vi "ManageInterfaces.vi"(0 "ClassWriterNative.lvclass":refnum<class "ClassWriterNative.lvclass">, 1 "ClassRef":refnum<vi>, 2 "HandleInterfacesData":T1, 5 "error in (no error)":errorcluster) -> (14 "ClassWriterNative.lvclass":refnum<class "ClassWriterNative.lvclass">, 19 "error out":errorcluster)   [LabVIEW 2020, in "ClassWriterNative.lvclass"]
uses:
  ClassWriterNative.lvclass
  C:/Program Files (x86)/National Instruments/LabVIEW 2020/resource/Framework/Providers/Open_GDS/ClassProviders/Provider_BaseClassInterface/ClassWriter_class/ClassWriter.lvclass
  Provider_BaseClassInterface/ClassWriter_class/HandleInterfacesData.ctl
  662f421e-4c37-4cdf-a30f-b2e85ba611a1.vi
  Common/InterfaceLibrary/InterfaceLibrary.lvlib
  Provider_BaseClassInterface/ClassWriter_class/ClassWriter.lvclass
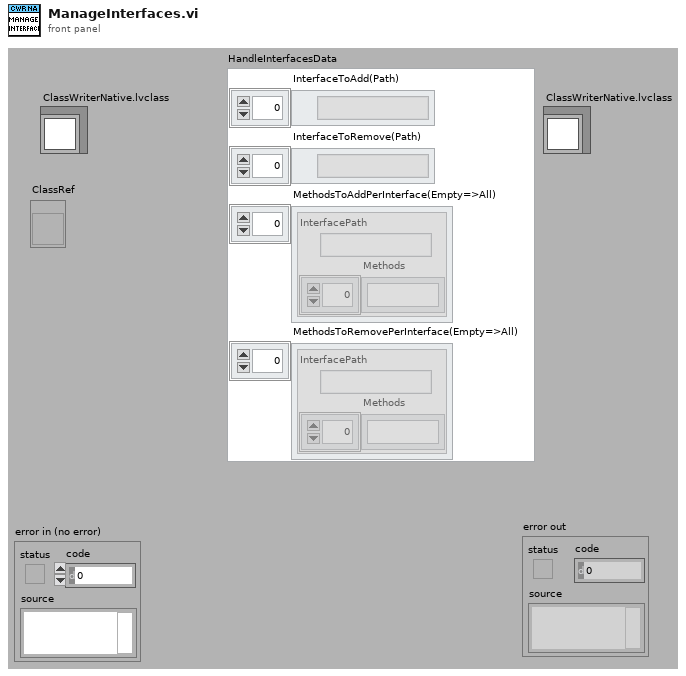
[diagram p1: front panel]
types:
  T1 = typedef "ClassWriter.lvclass/HandleInterfacesData.ctl" = cluster{"InterfaceToAdd(Path)":path[], "InterfaceToRemove(Path)":path[], "MethodsToAddPerInterface(Empty=>All)":cluster{"InterfacePath":path, "Methods":string[]}[], "MethodsToRemovePerInterface(Empty=>All)":cluster{"InterfacePath":path, "Methods":string[]}[]}
  T2 = cluster{"InterfacePath":path, "Methods":string[]}[]
  T3 = cluster{"InterfacePath":path, "Methods":string[]}
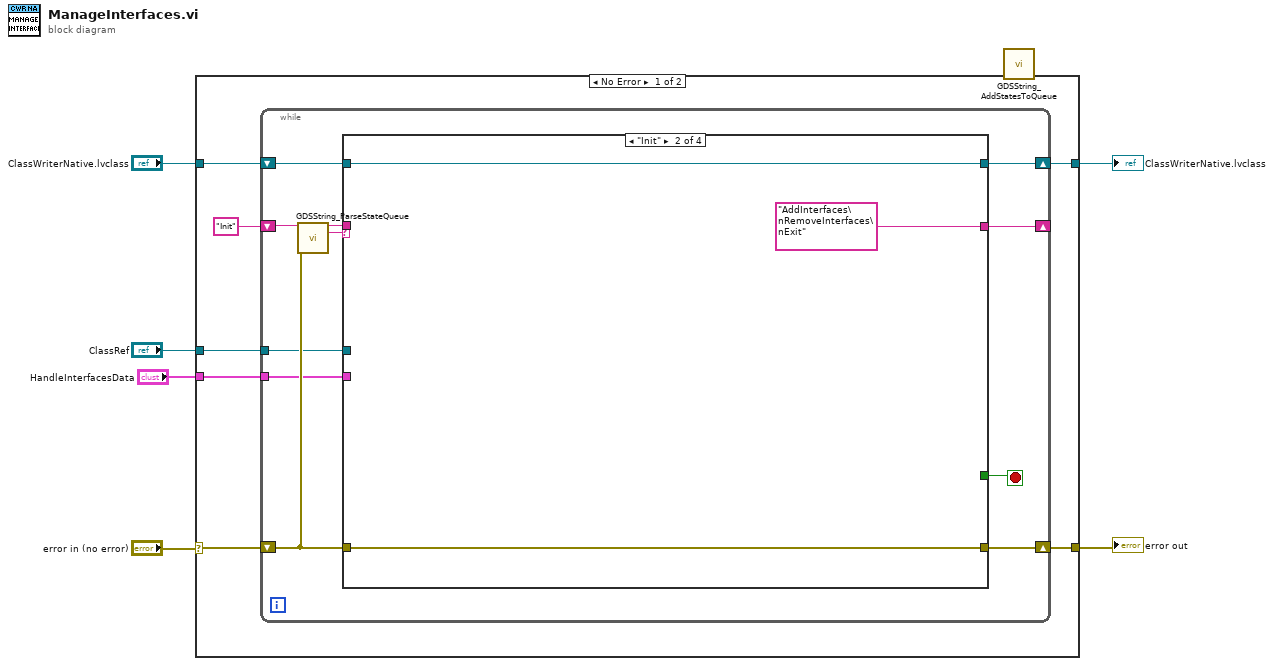
[diagram p0: block diagram]
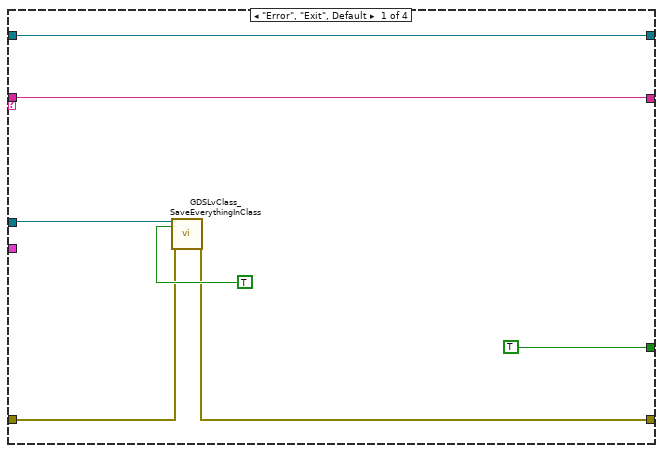
[diagram p2: hidden frame]
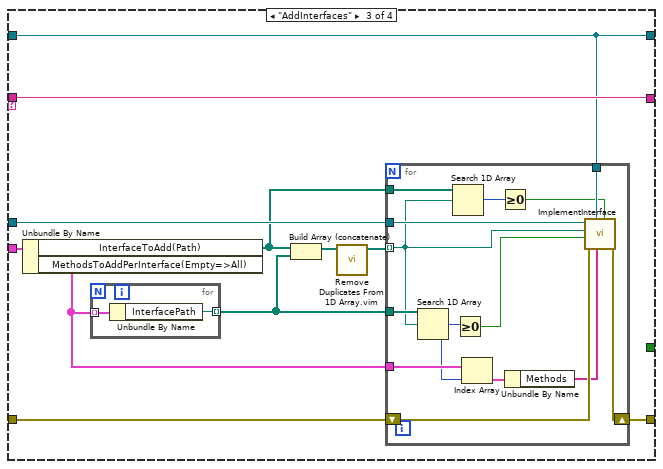
[diagram p3: hidden frame]
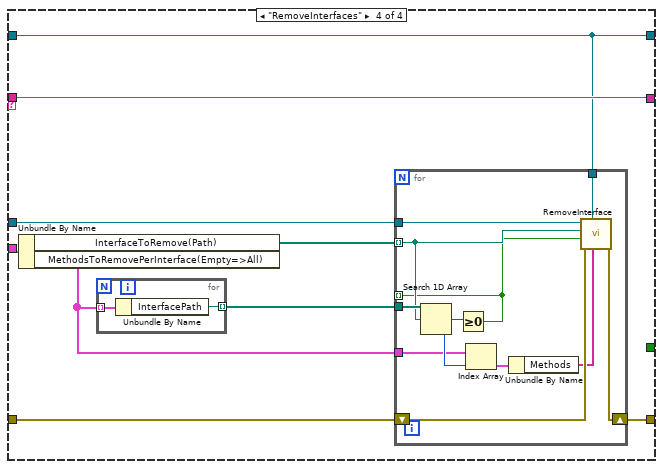
[diagram p4: hidden frame]
diagram:
  n1 = case shown="No Error" "error in (no error)" {
    selector: "error in (no error)" -> [w13 w84]
    tunnel: "ClassWriterNative.lvclass" -> [w9 w85]
    tunnel: [w12 w84] -> w5
    tunnel: [w8 w85] -> w4
    tunnel: "ClassRef" -> [w10 _]
    tunnel: "HandleInterfacesData" -> [w7 _]
    frame No Error {
      n2 = while {
        shift-right: [w20] -> w12
        shift-left: w13 -> [w21]
        shift-right: [w22] -> _
        shift-left: "Init" -> [w23]
        tunnel: w10 -> [w17]
        shift-right: [w15] -> w8
        shift-left: w9 -> [w16]
        tunnel: w7 -> [w14]
        stop <- w18 stop-if-true
        n3 = call "GDSString_ParseStateQueue.vi"("State Queue"=w23, "Error In (no error)"=w21) -> ("Remaining States"=w19:string, "Current State"=w24:string)  [unwired: 9 in, 3 out]
        n4 = case shown="\"Init\"" w24 {
          tunnel: [w31 "AddInterfaces\nRemoveInterfaces\nExit" w45 w70] -> w22
          tunnel: w21 -> [w25 w33 w43 w68]
          tunnel: [w26 w33 w42 w67] -> w20
          tunnel: w19 -> [w31 _ w45 w70]
          tunnel: [TRUE _ _ _] -> w18
          tunnel: w17 -> [w27 _ w44 w69]
          tunnel: w16 -> [w29 w32 w41 w66]
          tunnel: [w29 w32 w41 w66] -> w15
          tunnel: w14 -> [_ _ w40 w65]
          frame "Error", "Exit", Default {
            n5 = call "GDSLvClass_SaveEverythingInClass.vi"("ClassRefIn"=w27, "ForceResaving(False)"=TRUE, "error in"=w25) -> ("error out"=w26:errorcluster)  [unwired: 15 in, 1 out]
          }
          frame "Init" {
          }
          frame "AddInterfaces" {
            n6 = Unbundle By Name(w40) -> ("InterfaceToAdd(Path)"=w35:path[], "MethodsToAddPerInterface(Empty=>All)"=w39:T2)
            n7 = for {
              tunnel: w39 -> [w47] mode=indexing
              tunnel: [w46] -> w38 mode=indexing
              n8 = Unbundle By Name(w47) -> ("InterfacePath"=w46:path)
            }
            n9 = Build Array (concatenate)(w35, w38) -> (w37:path[])
            n10 = call "Remove Duplicates From 1D Array.vim"("array"=w37) -> ("array with duplicates removed"=w36:path[])  [unwired: 10 in]
            n11 = for {
              tunnel: w44 -> [w61]
              shift-right: [w59] -> w42
              shift-left: w43 -> [w60]
              tunnel: w41 -> [w58]
              tunnel: w36 -> [w51] mode=indexing
              tunnel: w38 -> [w57]
              tunnel: w39 -> [w55]
              tunnel: w35 -> [w48]
              n12 = Search 1D Array(1D array=w57, element=w51) -> (index of element=w54:i32)  [unwired: 1 in]
              n13 = Search 1D Array(1D array=w48, element=w51) -> (index of element=w49:i32)  [unwired: 1 in]
              n14 = Greater Or Equal To 0?(x=w54) -> (x >= 0?=w56:bool)
              n15 = Index Array(array=w55, index=w54) -> (element=w53:T3)
              n16 = Greater Or Equal To 0?(x=w49) -> (x >= 0?=w50:bool)
              n17 = Unbundle By Name(w53) -> ("Methods"=w52:string[])
              n18 = call "ImplementInterface.vi"("AddInterfaceToClass(If not you still might want to create methods)"=w50, "InterfaceMethodsToCreate"=w52, "ClassWriter.lvclass"=w58, "error in"=w60, "CreateMethods"=w56, "Interface Path"=w51, "LvClassPath/LvClassProjectItem"=w61) -> ("error out"=w59:errorcluster)  [unwired: 4 in]
            }
          }
          frame "RemoveInterfaces" {
            n19 = Unbundle By Name(w65) -> ("InterfaceToRemove(Path)"=w64:path[], "MethodsToRemovePerInterface(Empty=>All)"=w62:T2)
            n20 = for {
              tunnel: w62 -> [w72] mode=indexing
              tunnel: [w71] -> w63 mode=indexing
              n21 = Unbundle By Name(w72) -> ("InterfacePath"=w71:path)
            }
            n22 = for {
              tunnel: w69 -> [w83]
              shift-right: [w81] -> w67
              shift-left: w68 -> [w82]
              tunnel: w66 -> [w80]
              tunnel: [w73] -> _ mode=indexing
              tunnel: w64 -> [w76] mode=indexing
              tunnel: w63 -> [w77]
              tunnel: w62 -> [w75]
              n23 = Search 1D Array(1D array=w77, element=w76) -> (index of element=w79:i32)  [unwired: 1 in]
              n24 = Greater Or Equal To 0?(x=w79) -> (x >= 0?=w73:bool)
              n25 = Index Array(array=w75, index=w79) -> (element=w78:T3)
              n26 = Unbundle By Name(w78) -> ("Methods"=w74:string[])
              n27 = call "RemoveInterface.vi"("InterfaceMethodsToRemove"=w74, "ClassWriter.lvclass"=w80, "error in"=w82, "RemoveMethods"=w73, "Interface Path"=w76, "LvClassPath/LvClassProjectItem"=w83) -> ("error out"=w81:errorcluster)  [unwired: 5 in]
            }
          }
        }
      }
    }
    frame Error {
    }
  }
  "ClassWriterNative.lvclass" <- w4
  "error out" <- w5
  n28 = call "GDSString_AddStatesToQueue.vi"() -> ()  [unwired: 15 in, 1 out]
